vi "DisplayLCD.vi"(8 "error in (no error)":errorcluster, 10 "Display string":string, 11 "SerialPortRef":T1) -> (0 "error out":errorcluster, 3 "SerialPortRef 2":T1)   [LabVIEW 2015]
uses:
  <vilib>/Rock Robotics/WPI/SerialPort/WPI_SerialPortRef.ctl
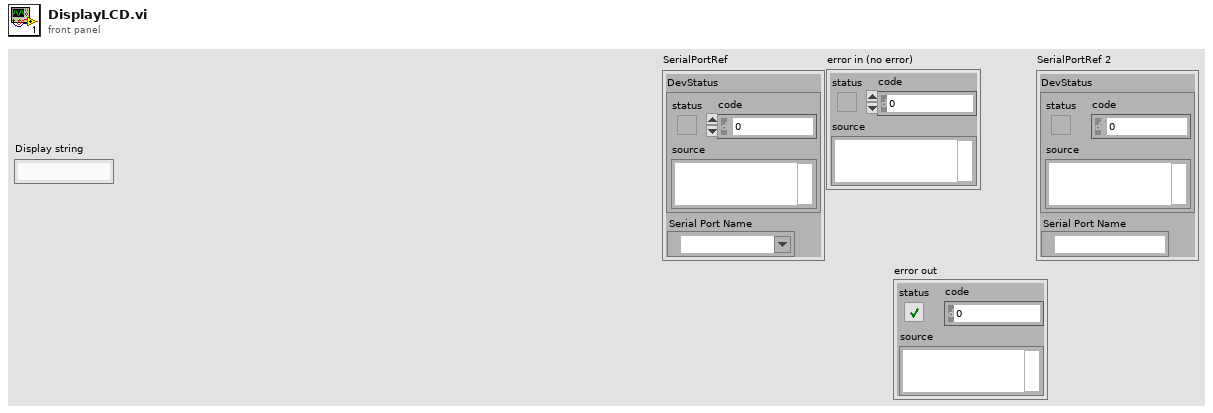
[diagram p1: front panel]
types:
  T1 = typedef "WPI_SerialPortRef.ctl" = cluster{"DevStatus":errorcluster, "Serial Port Name":refnum<visa-resource-name>}
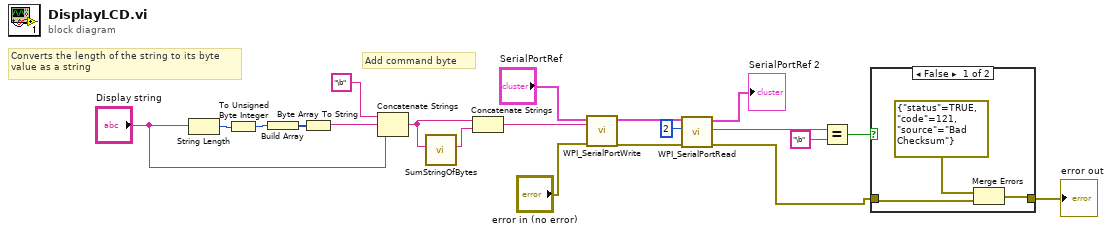
[diagram p0: block diagram]
diagram:
  # "Converts the length of the string to its byte \nvalue as a string"
  # "Add command byte"
  n1 = String Length(string="Display string") -> (length=w10:i32)
  n2 = To Unsigned Byte Integer(number=w10) -> (unsigned 8bit integer=w9:u8)
  n3 = Build Array(w9) -> (w8:u8[])
  n4 = Byte Array To String(unsigned byte array=w8) -> (string=w7:string)
  n5 = Concatenate Strings("\b" ("Buffer"), w7, "Display string") -> (w11:string)
  n6 = call "SumStringOfBytes.vi"("String Of Bytes"=w11) -> ("SumAsString"=w14:string)  [unwired: 10 in]
  n7 = Concatenate Strings(w11, w14) -> (w13:string)
  n8 = call <vilib>:"WPI_SerialPortWrite.vi"("error in (no error)"="error in (no error)", "Buffer"=w13, "SerialPortRef"="SerialPortRef") -> ("error out"=w17:errorcluster, "SerialPortRef"=w18:T1)  [unwired: 6 in, 1 out]
  n9 = call <vilib>:"WPI_SerialPortRead.vi"("error in (no error)"=w17, "Num Bytes to Read"=u32 2, "SerialPortRef"=w18) -> ("error out"=w3:errorcluster, "Buffer"=w6:string, "SerialPortRef"=→"SerialPortRef 2":T1)  [unwired: 6 in]
  n10 = Equal?(x=w6, y="\b") -> (x = y?=w4:bool)
  n11 = case shown="False" w4 {
    tunnel: w3 -> [w22 w24]
    tunnel: [w23 w24] -> w2
    frame False {
      n12 = Merge Errors(errorcluster {"status"=TRUE, "code"=121, "source"="Bad Checksum"} ("error out"), w22) -> (w23:errorcluster)
    }
    frame True {
    }
  }
  "error out" <- w2
